vi "Test Coffee Shop Removed Customer is Cleared.vi"(8 "error in (no error)":errorcluster, 11 "Coffee Shop Test In":refnum<class "Coffee Shop Test.lvclass">=refnum) -> (0 "error out":errorcluster, 3 "Coffee Shop Test Out":refnum<class "Coffee Shop Test.lvclass">)   [LabVIEW 2020, in "Coffee Shop Test.lvclass"]
uses:
  Coffee Shop Test.lvclass
  Processes/Coffee Shop/Coffee Shop.lvclass
  <vilib>/Astemes/Triarc Framework/Process/Process.lvclass
  C:/Program Files (x86)/National Instruments/LabVIEW 2020/vi.lib/Astemes/Triarc Framework/Application/Application.lvclass
  C:/Program Files (x86)/National Instruments/LabVIEW 2020/vi.lib/Astemes/Triarc Framework/Process/Process.lvclass
  C:/Program Files (x86)/National Instruments/LabVIEW 2020/vi.lib/Astemes/Triarc Framework/Base/Base.lvclass
  C:/Program Files (x86)/National Instruments/LabVIEW 2020/vi.lib/Astemes/Triarc Framework/Error Handler Interface/Error Handler Interface.lvclass
  C:/Program Files (x86)/National Instruments/LabVIEW 2020/vi.lib/Astemes/Triarc Framework/Logging/Logging.lvclass
  C:/Program Files (x86)/National Instruments/LabVIEW 2020/vi.lib/Astemes/Triarc Framework/Async Handler/Async Handler.lvclass
  C:/git/astemes-triarc-examples/source/Coffee Shop/Processes/Coffee Shop/Coffee Shop.lvclass
  <vilib>/Astemes/Triarc Framework/Application/Application.lvclass
  <vilib>/Astemes/Triarc Framework/Process/Public/Lifecycle/Lifecycle State.ctl
  <vilib>/Astemes/LUnit/Test Case.lvclass
  C:/Program Files (x86)/National Instruments/LabVIEW 2020/vi.lib/Astemes/LUnit/Test Case.lvclass
  C:/Program Files (x86)/National Instruments/LabVIEW 2020/vi.lib/Astemes/LUnit/LUnit Runnable.lvclass
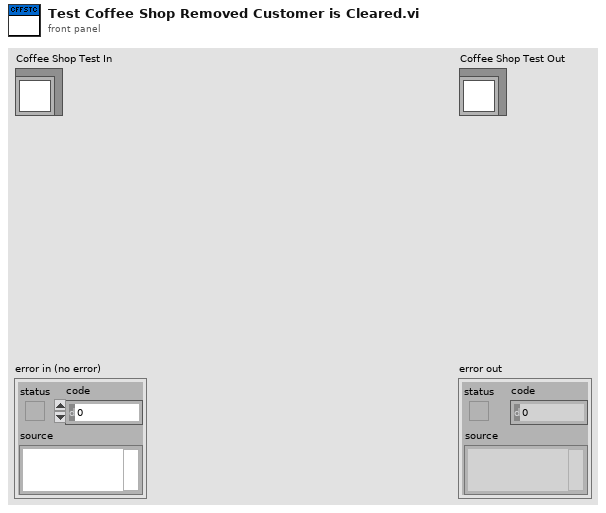
[diagram p1: front panel]
types:
  T1 = typedef "TF.lvlib/Process.lvclass/Lifecycle State.ctl" = enum16{"Uninitialized", "Initialized", "Started", "Running", "Stopped", "Finished"}
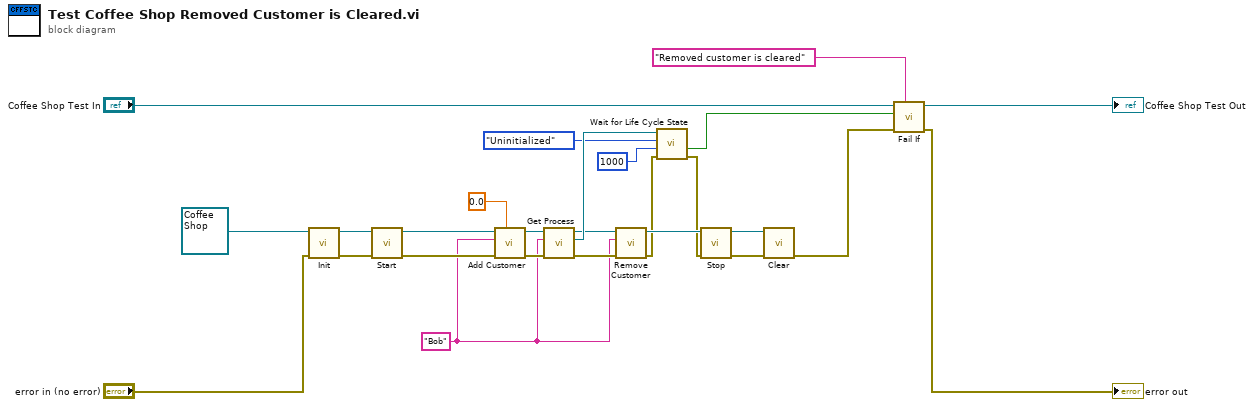
[diagram p0: block diagram]
diagram:
  w7 = "Bob" ("Name")
  n1 = call-dynamic "Init.vi"("error in (no error)"="error in (no error)", "Process In"=refnum<class "Coffee Shop.lvclass"> refnum ("Coffee Shop.lvclass")) -> ("error out"=w24:errorcluster, "Process Out"=w25:refnum<class "Coffee Shop.lvclass">)  [unwired: 8 in]
  n2 = call <vilib>:"Start.vi"("error in (no error)"=w24, "Process In"=w25) -> ("error out"=w19:errorcluster, "Process Out"=w18:refnum<class "Coffee Shop.lvclass">)  [unwired: 7 in, 1 out]
  n3 = call "Add Customer.vi"("Time scale [ms]"=0.0 ("Delay Before Leaving [s]"), "error in (no error)"=w19, "Name"=w7, "Coffee Shop in"=w18) -> ("error out"=w20:errorcluster, "Coffee Shop out"=w11:refnum<class "Coffee Shop.lvclass">)  [unwired: 6 in]
  n4 = call <vilib>:"Get Process.vi"("error in (no error)"=w20, "Process Name"=w7, "Application In"=w11) -> ("error out"=w12:errorcluster, "App Process"=w10:refnum<class "Process.lvclass">, "Application Out"=w9:refnum<class "Coffee Shop.lvclass">)  [unwired: 6 in]
  n5 = call "Remove Customer.vi"("error in (no error)"=w12, "Name"=w7, "Coffee Shop In"=w9) -> ("error out"=w6:errorcluster, "Coffee Shop Out"=w8:refnum<class "Coffee Shop.lvclass">)  [unwired: 7 in]
  n6 = call <vilib>:"Wait for Life Cycle State.vi"("error in (no error)"=w6, "timeout in ms (-1)"=1000, "Lifecycle State"=Lifecycle_State."Uninitialized", "Process In"=w10) -> ("error out"=w5:errorcluster, "timed out?"=w2:bool)  [unwired: 5 in, 1 out]
  n7 = call <vilib>:"Stop.vi"("error in (no error)"=w5, "Process In"=w8) -> ("error out"=w22:errorcluster, "Process Out"=w23:refnum<class "Coffee Shop.lvclass">)  [unwired: 7 in, 1 out]
  n8 = call-dynamic "Clear.vi"("error in (no error)"=w22, "Application In"=w23) -> ("error out"=w15:errorcluster)  [unwired: 9 in]
  n9 = call <vilib>:"Fail If.vi"("Description"="Removed customer is cleared", "error in (no error)"=w15, "Fail?"=w2, "LUnit Test Case In"="Coffee Shop Test In") -> ("error out"=→"error out":errorcluster, "LUnit Test Case Out"=→"Coffee Shop Test Out":refnum<class "Test Case.lvclass">)  [unwired: 6 in]
